vi "Turning with the Limelight.vi"() -> (0 "TurnCommand":dbl(knob)=nan scale=-1.0..1.0, 1 "Speed Command":dbl(knob)=nan scale=-1.0..1.0, 3 "TargetValid":bool)   [LabVIEW 2019]
uses:
  Framework/Robot Global Data.vi
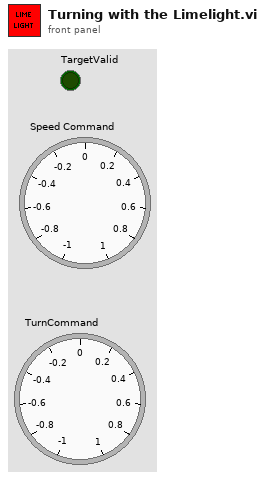
[diagram p1: front panel]
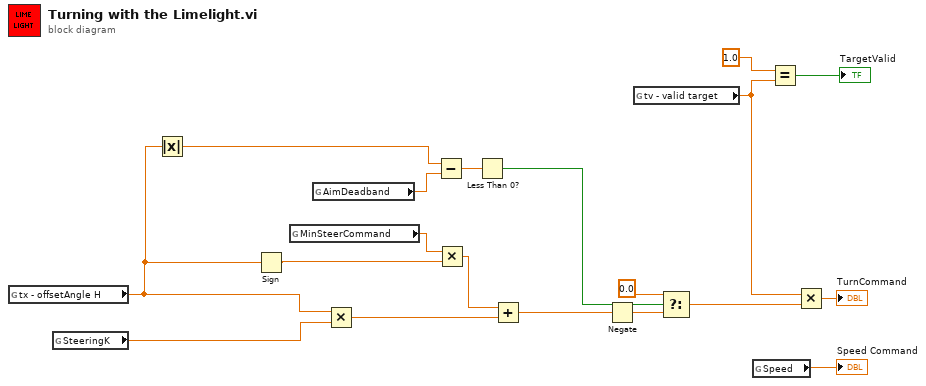
[diagram p0: block diagram]
diagram:
  n1 = global read "Robot Global Data.vi" "tx - offsetAngle H"() -> (w7:dbl)
  n2 = global read "Robot Global Data.vi" "SteeringK"() -> (w5:dbl)
  n3 = Absolute Value(x=w7) -> (abs(x)=w16:dbl)
  n4 = Sign(1:w7) -> (0:w11:dbl)
  n5 = global read "Robot Global Data.vi" "MinSteerCommand"() -> (w3:dbl)
  n6 = global read "Robot Global Data.vi" "AimDeadband"() -> (w4:dbl)
  n7 = Multiply(x=w7, y=w5) -> (x*y=w14:dbl)
  n8 = Subtract(x=w16, y=w4) -> (x-y=w17:dbl)
  n9 = Multiply(x=w3, y=w11) -> (x*y=w15:dbl)
  n10 = Less Than 0?(x=w17) -> (x < 0?=w18:bool)
  n11 = Add(x=w15, y=w14) -> (x+y=w10:dbl)
  n12 = Negate(x=w10) -> (-x=w2:dbl)
  n13 = global read "Robot Global Data.vi" "tv - valid target"() -> (w6:dbl)
  n14 = Select(t=0.0, s=w18, f=w2) -> (s? t:f=w13:dbl)
  n15 = global read "Robot Global Data.vi" "Speed"() -> (→"Speed Command":dbl)
  n16 = Equal?(x=1.0, y=w6) -> (x = y?=→"TargetValid":bool)
  n17 = Multiply(x=w6, y=w13) -> (x*y=→"TurnCommand":dbl)
